vi "Request.vi"(8 "error in (no error)":errorcluster, 9 "Device and Axis":string, 10 "Command String":string, 11 "VISA resource name":refnum<visa-resource-name>) -> (0 "error out":errorcluster, 1 "Response Bundle Array":T2(array[cluster]), 2 "Response String Array":string[](array[string]), 3 "VISA resource name out":refnum<visa-resource-name>, 4 "First Response Bundle":T1, 5 "Number of Replies":i32)   [LabVIEW 2020, in "Zaber A Series.lvlib"]
doc: "Writes a string to the serial port and then waits for all of the responses to be received. For inputting the command, it combines the Device and Axis input, Command List input, and Data value input to create a complete command. You could optionally send the complete command directly to the Command List input. Omitting the Device and Axis will send the command to all devices/axes. \n\nYou can use the All Commands or Basic Commands controls for the Command List input to easily select from the list of available commands. For getting or changing settings (get and set commands), you can also use the All Settings and Basic Settings controls as the data input. \n\nThe Enumerate VI is designed to provide an easy list of valid Device and Axis inputs. \n\nAn array containing the complete strings of the responses is returned on the Response String Array output, and the details of the format of the response are described here: http://www.zaber.com/wiki/Manuals/ASCII_Protocol_Manual#Replies. This VI also parses the strings, bundles the components, and returns them as an array of bundles on the Response Bundle Array pin. Additionally a pin returns the number of responses received. \n\nThis VI requires that the Initialize VI has been called with the same serial port."
uses:
  Zaber A Series.lvlib
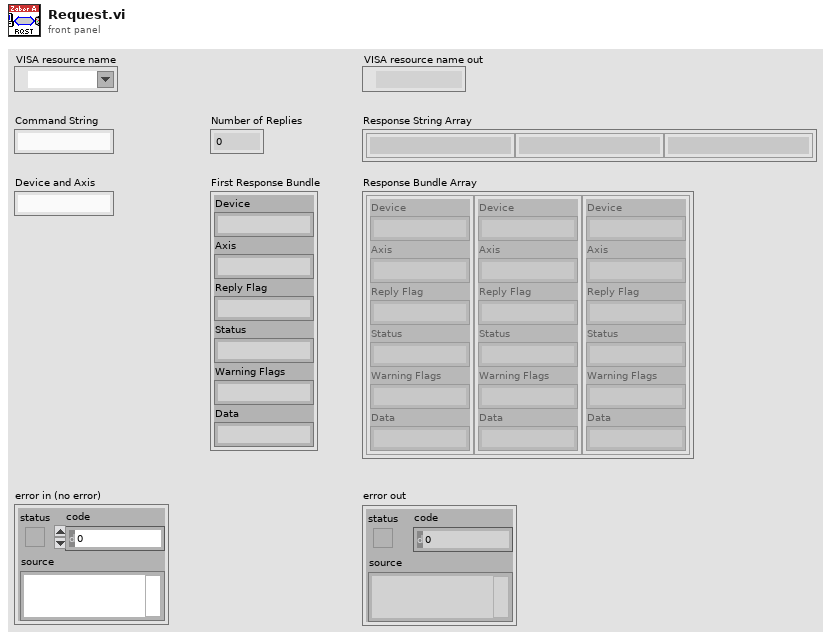
[diagram p1: front panel]
types:
  T1 = cluster{"Device":string, "Axis":string, "Reply Flag":string, "Status":string, "Warning Flags":string, "Data":string}
  T2 = cluster{"Device":string, "Axis":string, "Reply Flag":string, "Status":string, "Warning Flags":string, "Data":string}[]
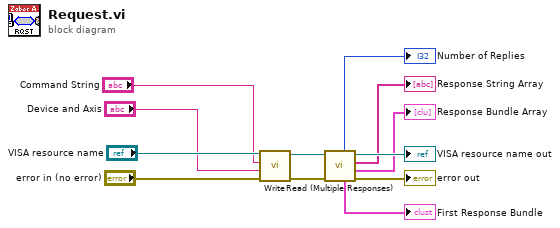
[diagram p0: block diagram]
diagram:
  n1 = call "Write.vi"("error in (no error)"="error in (no error)", "Device and Axis"="Device and Axis", "Command"="Command String", "VISA resource name"="VISA resource name") -> ("error out"=w2:errorcluster, "VISA resource name out"=w3:refnum<visa-resource-name>)  [unwired: 6 in]
  n2 = call "Read (Multiple Responses).vi"("error in (no error)"=w2, "VISA resource name"=w3) -> ("error out"=→"error out":errorcluster, "Response Bundle Array"=→"Response Bundle Array":T2, "Response String Array"=→"Response String Array":string[], "VISA resource name out"=→"VISA resource name out":refnum<visa-resource-name>, "First Response Bundle"=→"First Response Bundle":T1, "Number of Replies"=→"Number of Replies":i32)  [unwired: 4 in]
